vi "kontrola hitrosti_prava.vi"() -> ()   [LabVIEW 2019]
uses:
  <vilib>/Analysis/NI_AALBase.lvlib
panel:
  in  "Način krmiljenja:\nNapetost/tok":bool
  in  "merjen tok":dbl(slide)=100.0 caption="Offset" scale=85.0..115.0
  in  "Tab Control 2":enum32{"Napetost", "Tok"}(tab)
  out "tabela vseh zajemov napetosti napetosti":dbl[][](array[numeric])
  out "tabela vseh zajemov toka":dbl[][](array[numeric])
  out "array std dev zadnjih zajemov":dbl[](array[numeric])
  in  "?":enum32{"Napetost", "Tok"}(tab)
  out "Chart zajema napetosti":dynamicdata(graph)=[{"t0"=timestamp(3658204058.656474 s since 1904-01-01), "dt"=0.2, "Y"=[0.712291142137789, 0.9439230945296406, 0.7681391622796979, 1.2643625543602655, 1.1670099946593424], "attributes"=variant("NI_ChannelName"=variant(string "Voltage"), "NI_UnitDescription"=variant(string "Volts"))}]
  out "Chart zajema toka":dynamicdata(graph)
  in  "Tab Control":enum32{"Chart napetost", "Chart Tok"}(tab)
  out "std dev merjene nap":dbl format="%0.2f"
  out "Chart std dev":dbl(graph)=0.5891997348288455
  out "chart povprecji":dbl(graph)=0.971145189593347
  out "trenutno povprecje":dbl format="%0.2f"
  in  "n-krat std dev":dbl=1.0
  out "?":bool[](array[boolean])
  in  "merjena napetost":dbl(slide)=15.0 caption="Amplitude" scale=13.5..16.5
  out "chart hitrosti":dbl(graph)=292.0
  in  "korak skoka hitrosti":dbl=1.0
  out "?":dbl(knob)=300.0 scale=250.0..350.0
  in  "zeljena napetost\nEksperimentalno določena":dbl=15.0
  out "array povprecji zadnjih zajemov":dbl[](array[numeric])
  out "array zadnjega zajema napetosti":dbl[](array[numeric])
  in  "stop":bool
  # "Povprečje in std dev se izračuna po vsakem zajemu (npr 10k samples). Če je vzorčenje 10ks/s, bo povprečje izračunano 1x na sekundo"
  # "MERJENA VREDNOST"
  # "POVPREČNA NAPETOST IN STD DEV"
  # "Hitrost pomika"
  # "HITROST"
  # "hitrost se vedno spremeni za enak, vnaprej določen korak"
  # "Hitrost se prilagodi če je povprečna izmerjena napetost manjša oz. večja od željene napetosti\n\nČe je izmerjena napetost enaka željeni +/- n-kratniku std. dev merjeni napetosti, se hitrost ne spremeni"
  # "ODLOČITVENA TABELA"
  # "1. Večja nap?"
  # "1"
  # "2"
  # "2. Enako +/- n-krat std dev ?"
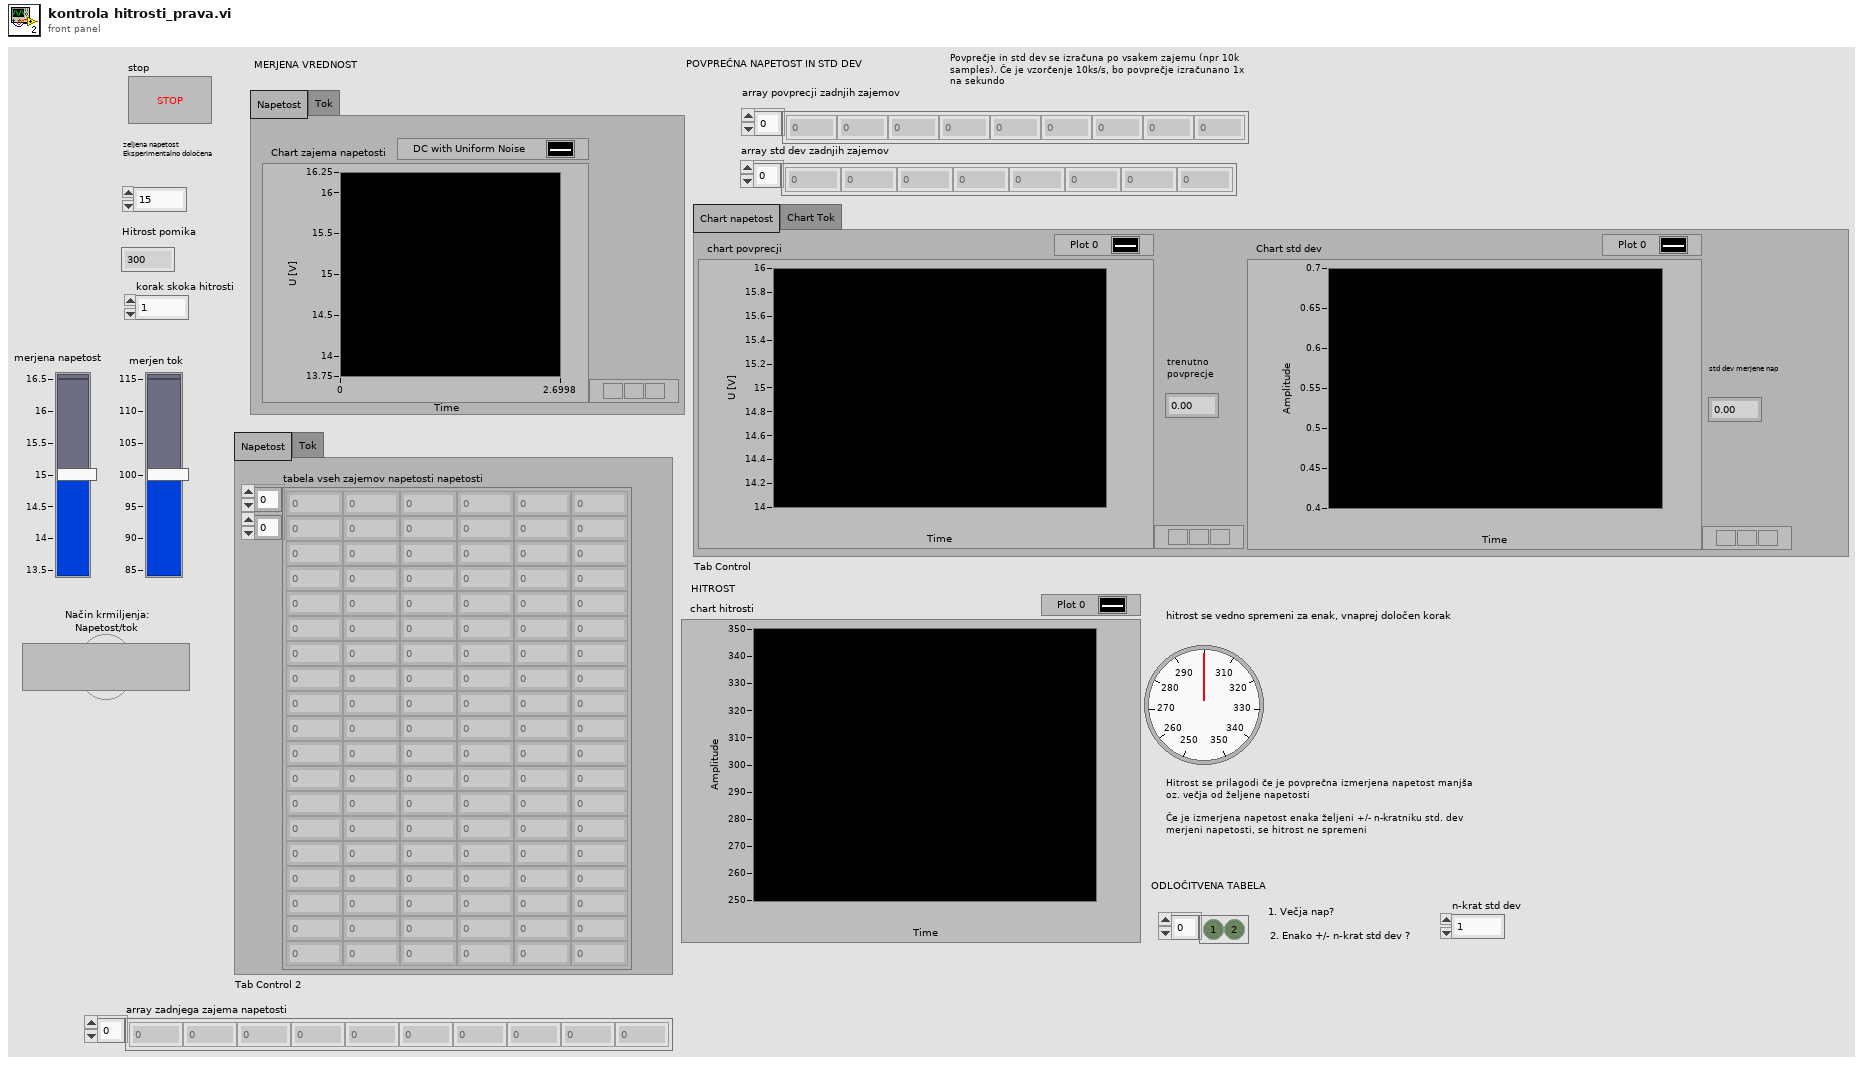
[diagram p1: front panel]
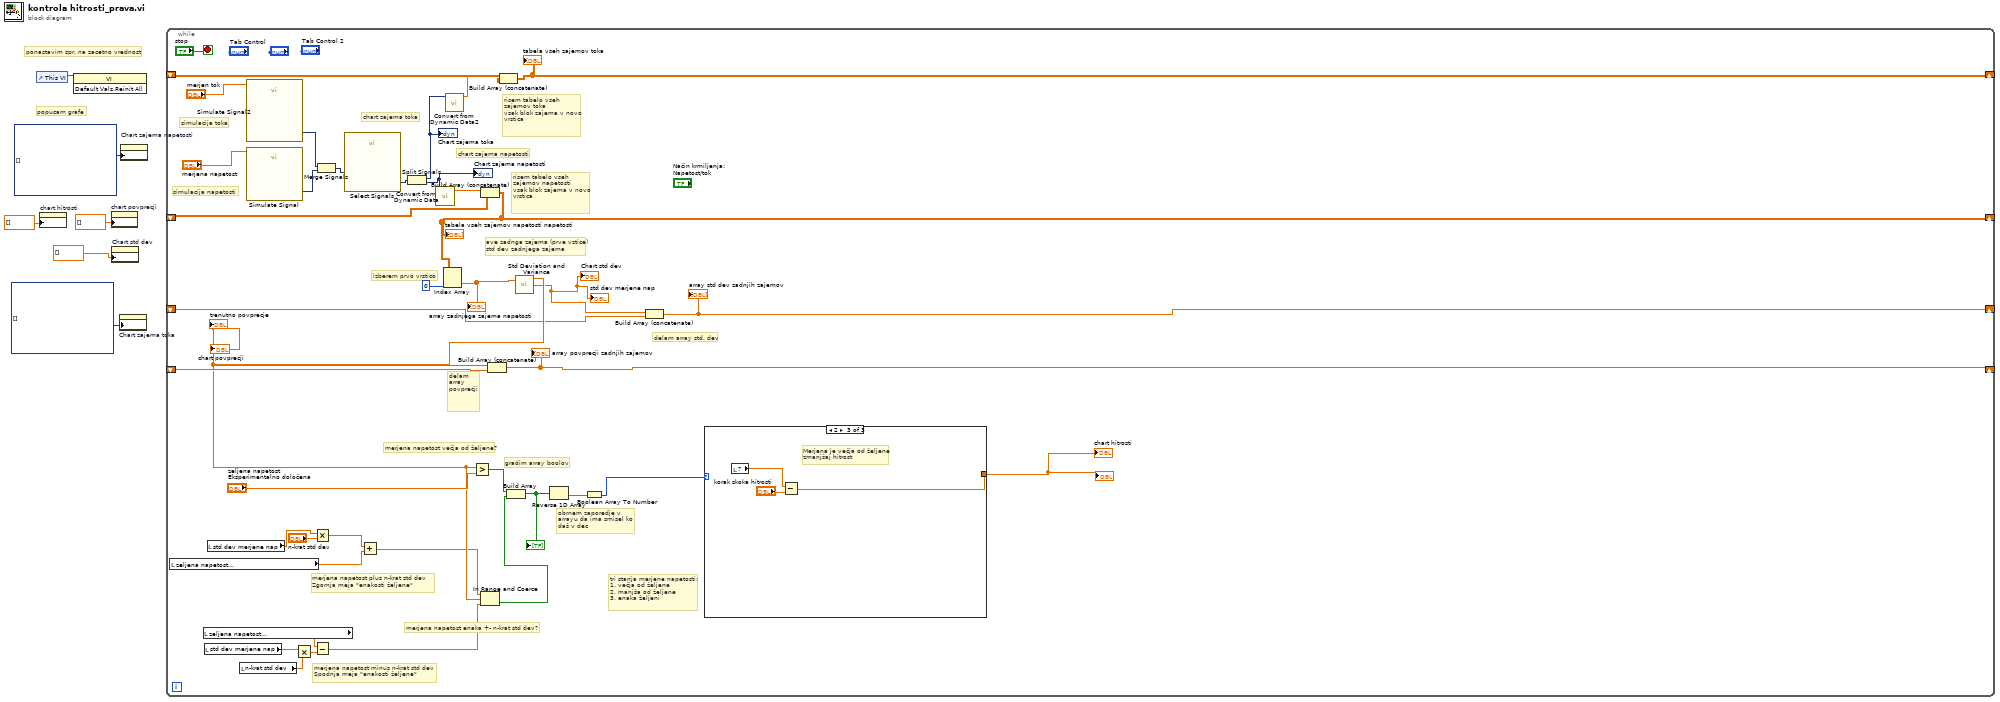
[diagram p0: block diagram]
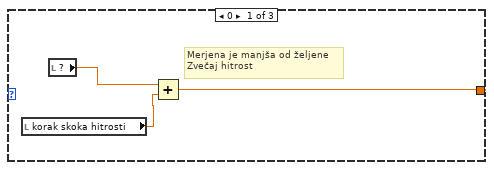
[diagram p2: hidden frame]
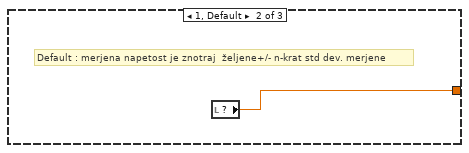
[diagram p3: hidden frame]
diagram:
  # "popucam grafe"
  # "ponastavim spr. na zacetno vrednost"
  n1 = control-ref of="This VI"() -> (w6:refnum<vi>)
  n2 = property on="chart hitrosti" class="WFChart (strict)"("History Data"=dbl[] []) -> ()  [unwired: 2 in, 2 out]
  n3 = invoke class="VI" method="Default Vals.Reinit All"(reference=w6) -> ()  [unwired: 2 in, 3 out]
  n4 = property on="chart povprecji" class="WFChart (strict)"("History Data"=dbl[] []) -> ()  [unwired: 2 in, 2 out]
  n5 = property on="Chart std dev" class="WFChart (strict)"("History Data"=dbl[] []) -> ()  [unwired: 2 in, 2 out]
  n6 = property on="Chart zajema toka" class="WFChart (strict)"("History Data"=dynamicdata[] []) -> ()  [unwired: 2 in, 2 out]
  n7 = property on="Chart zajema napetosti" class="WFChart (strict)"("History Data"=dynamicdata[] []) -> ()  [unwired: 2 in, 2 out]
  n8 = while {
    shift-right: [w40] -> _
    shift-left: _ -> [w39]
    shift-right: [w43] -> _
    shift-left: _ -> [w44]
    shift-right: [w19] -> _
    shift-left: _ -> [w18]
    shift-right: [w10] -> _
    shift-left: _ -> [w9]
    stop <- "stop" stop-if-true
    # "chart zajema toka"
    # "risem tabelo vseh zajemov toka\nvsak blok zajema v novo vrstica"
    # "simulacija napetosti"
    # "simulacija toka"
    # "delam array std. dev"
    # "tri stanja merjene napetosti:\n1. večja od željene\n2. manjša od željene\n3. enaka željeni"
    # "obrnem zaporedje v arrayu da ima smisel ko daš v dec"
    # "gradim array boolov"
    # "merjena napetost enaka +- n-krat std dev?"
    # "merjena napetost večja od željene?"
    # "merjena napetost plus n-krat std dev\nZgornja meja \"enakosti željene\""
    # "merjena napetost minus n-krat std dev\nSpodnja meja \"enakosti željene\""
    # "chart zajema napetosti"
    # "delam array povprecji"
    # "ave zadnga zajema (prve vstice)\nstd dev zadnjega zajema"
    # "risem tabelo vseh zajemov napetosti\nvsak blok zajema v novo vrstica"
    # "izberem prvo vrstico"
    n9 = local read "zeljena napetost\nEksperimentalno določena"() -> (w23:dbl)
    n10 = local read "zeljena napetost\nEksperimentalno določena"() -> (w29:dbl)
    n11 = local read "std dev merjene nap"() -> (w28:dbl)
    n12 = local read "std dev merjene nap"() -> (w25:dbl)
    n13 = local read "n-krat std dev"() -> (w20:dbl)
    n14 = call "Simulate Signal2"("Offset"="merjen tok") -> ("DC with Uniform Noise"=w15:dynamicdata)  [unwired: 13 in, 1 out]
    n15 = call "Simulate Signal"("Offset"="merjena napetost") -> ("DC with Uniform Noise"=w14:dynamicdata)  [unwired: 13 in, 1 out]
    n16 = Multiply(x=w28, y=w20) -> (x*y=w27:dbl)
    n17 = Multiply(x=w25, y="n-krat std dev") -> (x*y=w24:dbl)
    n18 = Subtract(x=w29, y=w27) -> (x-y=w26:dbl)
    n19 = Merge Signals(w15, w14) -> (w17:dynamicdata)
    n20 = call "Select Signals"("Signals"=w17) -> ("Signal Out"=w16:dynamicdata)  [unwired: 9 in, 1 out]
    n21 = Add(x=w24, y=w23) -> (x+y=w22:dbl)
    n22 = Split Signals(w16) -> (w12:dynamicdata, w13:dynamicdata)  [unwired: 2 in]
    "Chart zajema napetosti" <- w13
    "Chart zajema toka" <- w12
    n23 = call "Convert from Dynamic Data"("Dynamic Data Type"=w13) -> ("Array"=w41:dbl[])  [unwired: 3 in]
    n24 = call "Convert from Dynamic Data2"("Dynamic Data Type"=w12) -> ("Array"=w11:dbl[])  [unwired: 3 in]
    n25 = Build Array (concatenate)(w41, w39) -> (w40:dbl[][])
    "tabela vseh zajemov napetosti napetosti" <- w40
    n26 = Index Array(array=w40, index (row)=0) -> (element=w38:dbl[])  [unwired: 1 in]
    "array zadnjega zajema napetosti" <- w38
    n27 = Build Array (concatenate)(w11, w9) -> (w10:dbl[][])
    "tabela vseh zajemov toka" <- w10
    n28 = call <vilib>:"Std Deviation and Variance.vi"("X"=w38) -> ("mean"=w31:dbl, "standard deviation"=w8:dbl)  [unwired: 1 in, 1 out]
    "trenutno povprecje" <- w31
    "chart povprecji" <- w31
    "Chart std dev" <- w8
    "std dev merjene nap" <- w8
    n29 = Greater?(x=w31, y="zeljena napetost\nEksperimentalno določena") -> (0:w36:bool)
    n30 = In Range and Coerce(upper limit=w22, x=w31, lower limit=w26) -> (In Range?=w30:bool)  [unwired: 1 out]
    n31 = Build Array (concatenate)(w31, w44) -> (w43:dbl[])
    "array povprecji zadnjih zajemov" <- w43
    n32 = Build Array(w36, w30) -> (w35:bool[])
    "?" <- w35
    n33 = Reverse 1D Array(array=w35) -> (reversed array=w34:bool[])
    n34 = Boolean Array To Number(Boolean array=w34) -> (number=w33:u32)
    n35 = Build Array (concatenate)(w8, w18) -> (w19:dbl[])
    "array std dev zadnjih zajemov" <- w19
    n36 = case shown="2" w33 {
      tunnel: [w47 w50 w51] -> w42
      frame 0 {
        # "Merjena je manjša od željene \nZvečaj hitrost"
        n37 = local read "korak skoka hitrosti"() -> (w49:dbl)
        n38 = local read item#8() -> (w48:dbl)
        n39 = Add(x=w48, y=w49) -> (x+y=w47:dbl)
      }
      frame 1, Default {
        # "Default : merjena napetost je znotraj  željene+/- n-krat std dev. merjene"
        n40 = local read item#8() -> (w50:dbl)
      }
      frame 2 {
        # "Merjena je večja od željene\nzmanjšaj hitrost"
        n41 = local read item#8() -> (w52:dbl)
        n42 = Subtract(x=w52, y="korak skoka hitrosti") -> (x-y=w51:dbl)
      }
    }
    "?" <- w42
    "chart hitrosti" <- w42
  }
